vi "Get Input From Web.vi"() -> (3 "standard output":string)   [LabVIEW 2021]
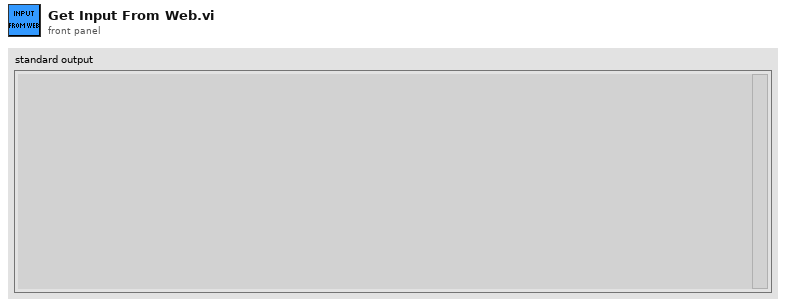
[diagram p1: front panel]
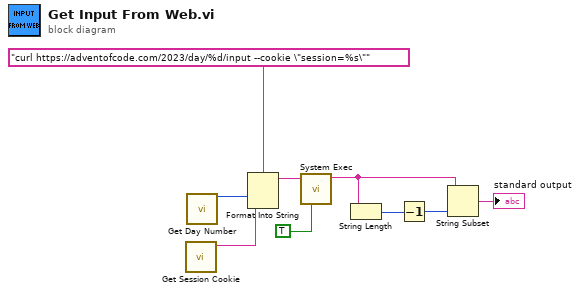
[diagram p0: block diagram]
diagram:
  n1 = call "Get Session Cookie.vi"() -> ("Session"=w6:string)  [unwired: 11 in]
  n2 = call "Get Day Number.vi"() -> ("Day"=w9:i32)  [unwired: 11 in]
  n3 = Format Into String(format string="curl https://adventofcode.com/2023/day/%d/input --cookie \"session=%s\"", w9, w6) -> (resulting string=w7:string)  [unwired: 2 in, 1 out]
  n4 = call <vilib>:"System Exec.vi"("run minimized? (F)"=TRUE, "command line"=w7) -> ("standard output"=w4:string)  [unwired: 6 in, 3 out]
  n5 = String Length(string=w4) -> (length=w5:i32)
  n6 = Decrement(x=w5) -> (x-1=w2:i32)
  n7 = String Subset(string=w4, length (rest)=w2) -> (substring=→"standard output":string)  [unwired: 1 in]
